vi "ClimberExtend.vi"(11 "Button":bool) -> ()   [LabVIEW 2015]
uses:
  <vilib>/Rock Robotics/WPI/Solenoid/Deprecated/WPI_SolenoidSetBool.vi
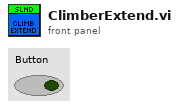
[diagram p1: front panel]
types:
  T1 = typedef "WPI_SolenoidDevRef.ctl" = cluster{"DevStatus":errorcluster, "Pneumatics Control Module":u8, "Forward Solenoid Channel":T2, "Reverse Solenoid Channel":T2}
  T2 = typedef "WPI_SolenoidChannel.ctl" = enum8{"Solenoid 0", "Solenoid 1", "Solenoid 2", "Solenoid 3", "Solenoid 4", "Solenoid 5", "Solenoid 6", "Solenoid 7", "Invalid"}
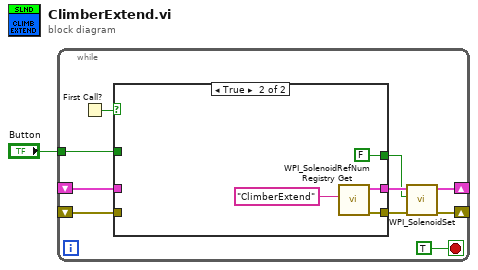
[diagram p0: block diagram]
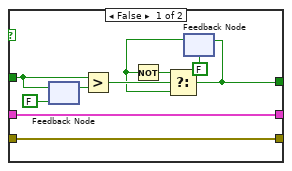
[diagram p2: hidden frame]
diagram:
  n1 = while {
    shift-right: [w8] -> _
    shift-left: _ -> [w4]
    shift-right: [w9] -> _
    shift-left: _ -> [w5]
    tunnel: "Button" -> [w3]
    stop <- TRUE stop-if-true
    n2 = First Call?() -> (First Call?: T/F=w6:bool)
    n3 = case shown="True" w6 {
      tunnel: [w21 w24] -> w11
      tunnel: [w20 w23] -> w10
      tunnel: [w12 FALSE] -> w7
      tunnel: w5 -> [w21 _]
      tunnel: w4 -> [w20 _]
      tunnel: w3 -> [w17 _]
      frame False {
        n4 = feedback-in #1(w17) -> ()
        n5 = feedback #1(FALSE ("Button")) -> (w18:bool)
        n6 = Greater?(x=w17, y=w18) -> (0:w16:bool)
        n7 = feedback #2(FALSE) -> (w13:bool)
        n8 = Not(x=w13) -> (.not. x?=w14:bool)
        n9 = Select(t=w14, s=w16, f=w13) -> (s? t:f=w12:bool)
        n10 = feedback-in #2(w12) -> ()
      }
      frame True {
        n11 = call <vilib>:"WPI_SolenoidRefNum Registry Get.vi"("refnum name"="ClimberExtend") -> ("error out"=w23:errorcluster, "SolenoidDevRef"=w24:T1)  [unwired: 9 in]
      }
    }
    n12 = call-poly <vilib>:"WPI_SolenoidSet.vi"("error in (no error)"=w10, "Value"=w7, "SolenoidDevRef"=w11) -> ("error out"=w8:errorcluster, "SolenoidDevRef"=w9:T1)  [unwired: 7 in]
  }
